vi "close.vi"(8 "error in":errorcluster, 11 "module in":refnum<class "Watchdog runtime.lvclass">) -> (0 "error out":errorcluster)   [LabVIEW 2013, in "Watchdog runtime.lvclass"]
doc: "Provides an interface for terminating a module instance. While this interface performs no operations, a child should close and deallocate any open references or memory."
uses:
  Watchdog runtime.lvclass
  <vilib>/NI/Tag Bus Data Framework/fixed module parent/module/execution/fixed channel runtime.lvclass
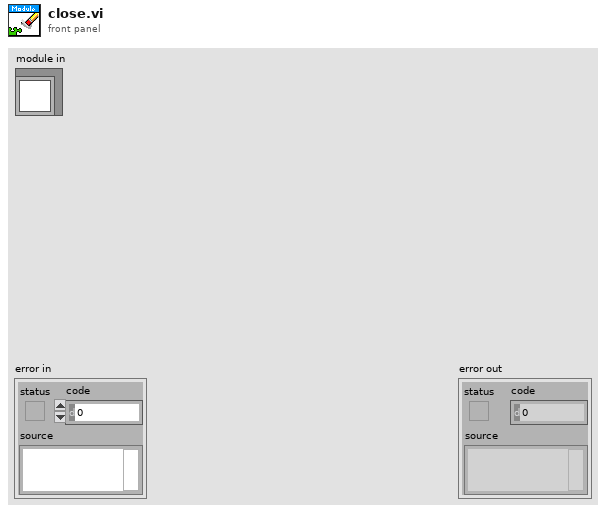
[diagram p1: front panel]
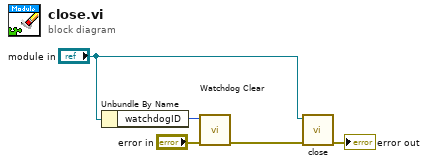
[diagram p0: block diagram]
diagram:
  n1 = Unbundle By Name("module in") -> ("watchdogID"=w3:u32)
  n2 = call <vilib>:"Watchdog Clear.vi"("error in (no error)"="error in", "watchdogID in"=w3) -> ("error out"=w2:errorcluster)  [unwired: 5 in]
  n3 = call-parent "close.vi"("error in"=w2, "module in"="module in") -> ("error out"=→"error out":errorcluster)  [unwired: 9 in]
